vi "Hopper Lift Motor Control.vi"(1 "Floor Position":dbl, 2 "Full Up Button":bool, 3 "Floor Button":bool, 4 "Unload Position":dbl, 5 "Unload Button":bool, 6 "Full Up Position":dbl) -> (0 "New Position":i32)   [LabVIEW 2019]
uses:
  Variables/Hopper Position Variable.vi
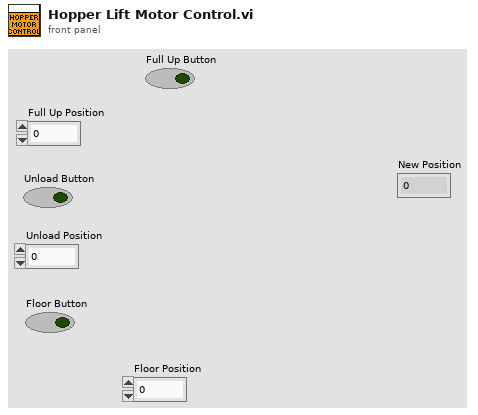
[diagram p1: front panel]
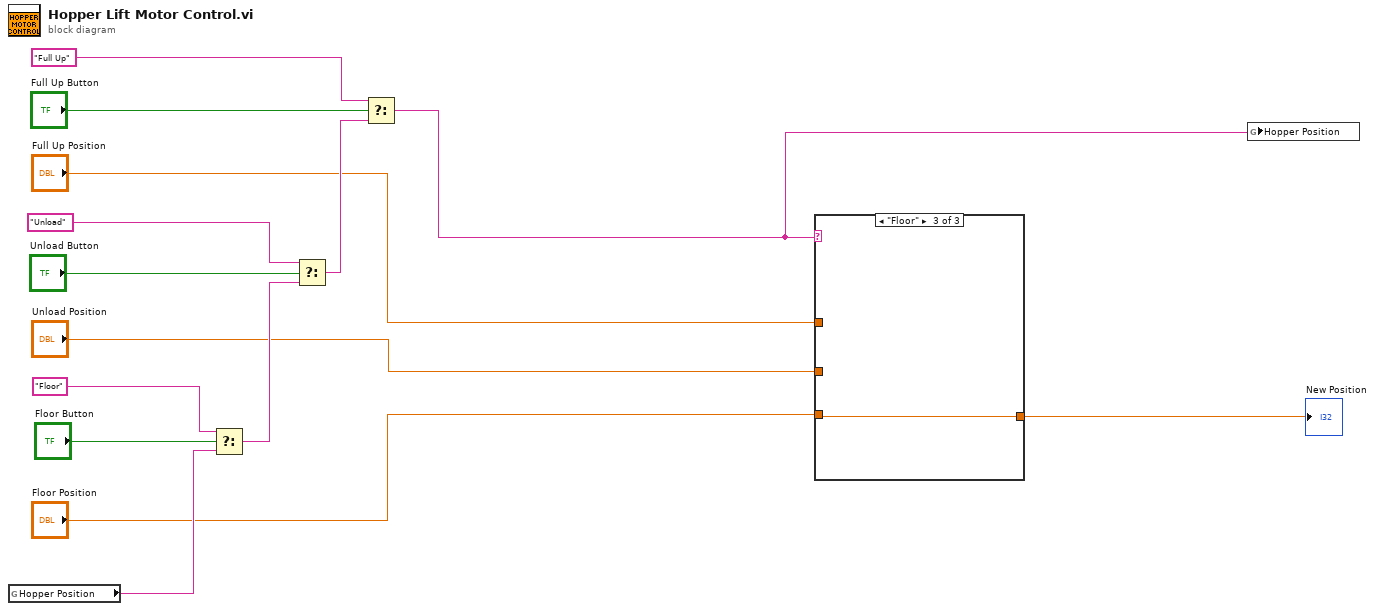
[diagram p0: block diagram]
diagram:
  n1 = global read "Hopper Position Variable.vi" "Hopper Position"() -> (w13:string)
  n2 = Select(t="Floor", s="Floor Button", f=w13) -> (s? t:f=w14:string)
  n3 = Select(t="Unload", s="Unload Button", f=w14) -> (s? t:f=w6:string)
  n4 = Select(t="Full Up", s="Full Up Button", f=w6) -> (s? t:f=w4:string)
  n5 = case shown="\"Floor\"" w4 {
    tunnel: [w15 w16 w17] -> w5
    tunnel: "Full Up Position" -> [w15 _ _]
    tunnel: "Unload Position" -> [_ w16 _]
    tunnel: "Floor Position" -> [_ _ w17]
    frame "Full Up", Default {
    }
    frame "Unload" {
    }
    frame "Floor" {
    }
  }
  "New Position" <- w5
  n6 = global write "Hopper Position Variable.vi" "Hopper Position"(w4) -> ()
